vi "polling_mc.vi"() -> ()   [LabVIEW 2013, in "AvaSpec.lvlib" / "Avantes Spectrometer Functions.lvlib"]
uses:
  Avantes Spectrometer Functions.lvlib
  Instance          14 18Saved   polling_mc .vi
  Instance          13 18Saved   polling_mc .vi
  Instance          12 18Saved   polling_mc .vi
  Instance          10 18Saved   polling_mc .vi
  Instance           9 18Saved   polling_mc .vi
  Instance           8 18Saved   polling_mc .vi
panel:
  in  "a_pMeasConfig2":T1={"StartPixel"=0, "StopPixel"=0, "IntTime"=25.0, "IntDelay"=0, "NrOfAVG"=1, "DarkEnable"=0, "ForgetPercentage"=0, "SmoothPix"=0, "SmoothModel"=0, "SatDetection"=0, "TriggerMode"=0, "TriggerSource"=0, "TriggerSourceType"=0, "FlashesPerScan"=0, "LaserDelay"=0, "LaserWidth"=0, "LaserWavelenght"=0.0, "RamSpectra"=0}
  in  "a_pMeasConfig1":T1={"StartPixel"=0, "StopPixel"=0, "IntTime"=25.0, "IntDelay"=0, "NrOfAVG"=1, "DarkEnable"=0, "ForgetPercentage"=0, "SmoothPix"=0, "SmoothModel"=0, "SatDetection"=0, "TriggerMode"=0, "TriggerSource"=0, "TriggerSourceType"=0, "FlashesPerScan"=0, "LaserDelay"=0, "LaserWidth"=0, "LaserWavelenght"=0.0, "RamSpectra"=0}
  out "a_pNumPixels2":u16
  out "a_pNumPixels":u16
  in  "Sync Master":enum32{"Top Master", "Bottom Master"}(radio)
  in  "Sync Mode":enum32{"SyncMode On", "Sync Mode Off"}(radio)
  out "Serial2":string
  out "Serial1":string
  out "AVS_StopMeasure2":i32
  out "AVS_Deactivate2":i32
  out "Scope Values 2":cluster{"Y":dbl[], "Y":dbl[]}[](graph)
  out "a_pTimeLabel2":u32
  out "a_pDeviceId2":u8[](array[numeric])
  out "Handle2":i32
  out "Scope Values":cluster{"Y":dbl[], "Y":dbl[]}[](graph)
  out "a_pTimeLabel1":u32
  out "AVS_StopMeasure":i32
  out "AVS_Done":i32
  out "AVS_Deactivate":i32
  in  "Exit":bool
  in  "Stop":bool
  out "Handle1":i32
  out "a_pDeviceId1":u8[](array[numeric])
  in  "Start":bool
  in  "a_hWnd":i32
  out "Port":i32
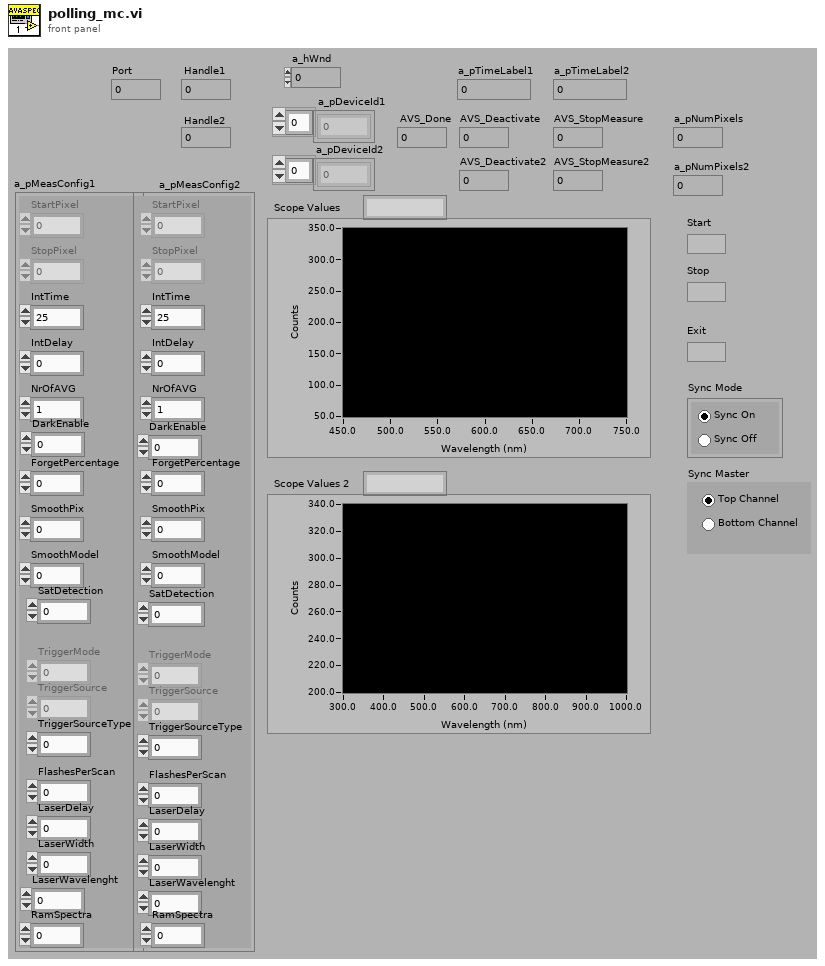
[diagram p1: front panel]
types:
  T1 = cluster{"StartPixel":u16, "StopPixel":u16, "IntTime":sgl, "IntDelay":u32, "NrOfAVG":u32, "DarkEnable":u8, "ForgetPercentage":u8, "SmoothPix":u16, "SmoothModel":u8, "SatDetection":u8, "TriggerMode":u8, "TriggerSource":u8, "TriggerSourceType":u8, "FlashesPerScan":u16, "LaserDelay":u32, "LaserWidth":u32, "LaserWavelenght":sgl, "RamSpectra":u16}
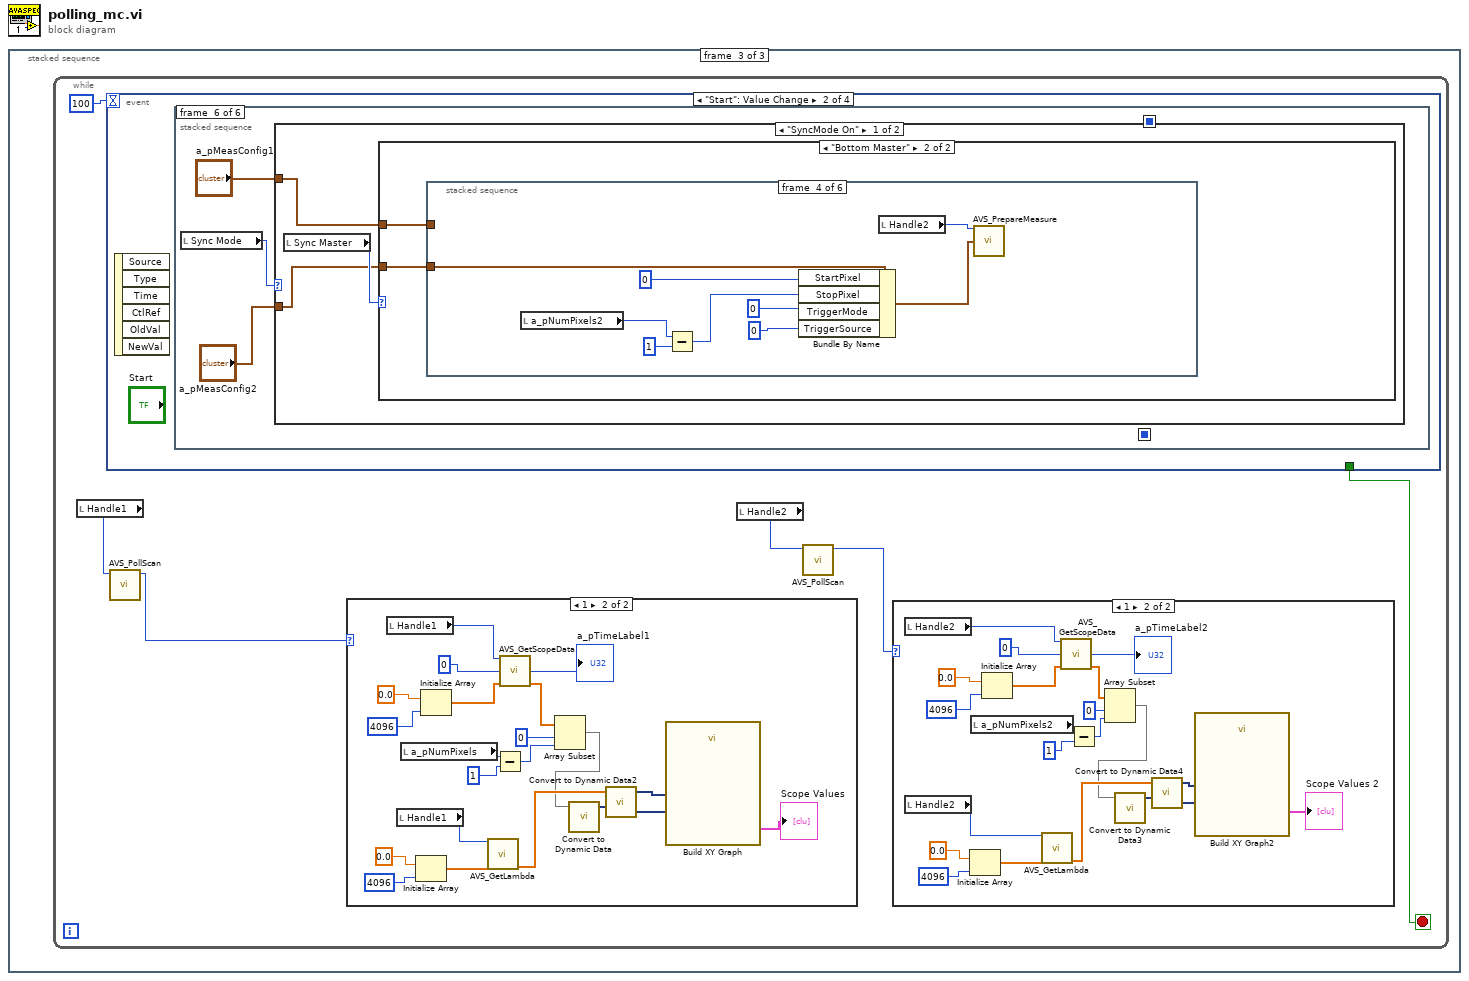
[diagram p0: block diagram]
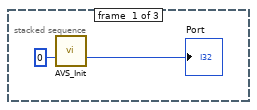
[diagram p2: hidden frame]
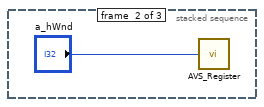
[diagram p3: hidden frame]
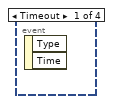
[diagram p6: hidden frame]
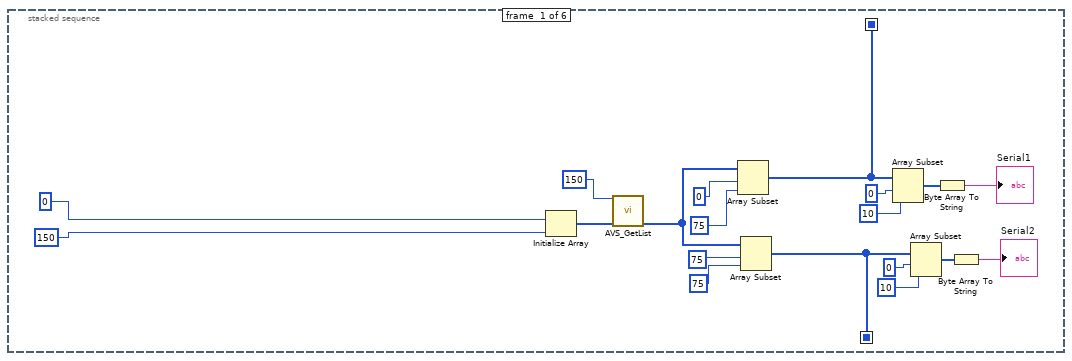
[diagram p7: hidden frame]
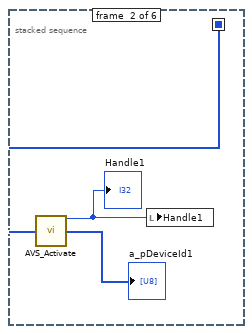
[diagram p8: hidden frame]
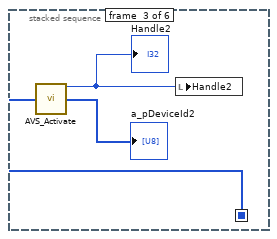
[diagram p9: hidden frame]
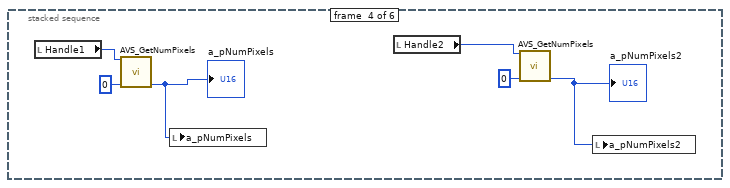
[diagram p10: hidden frame]
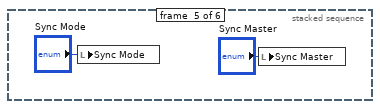
[diagram p11: hidden frame]
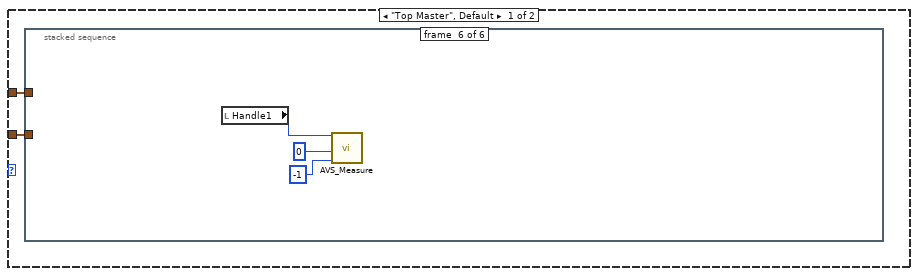
[diagram p12: hidden frame]
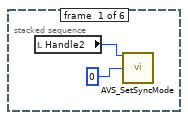
[diagram p13: hidden frame]
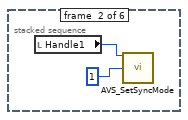
[diagram p14: hidden frame]
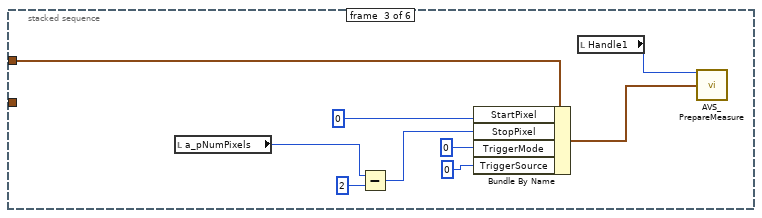
[diagram p15: hidden frame]
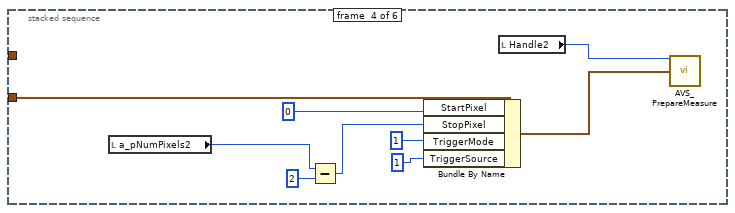
[diagram p16: hidden frame]
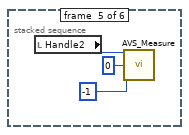
[diagram p17: hidden frame]
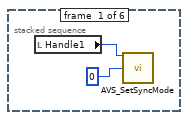
[diagram p18: hidden frame]
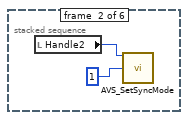
[diagram p19: hidden frame]
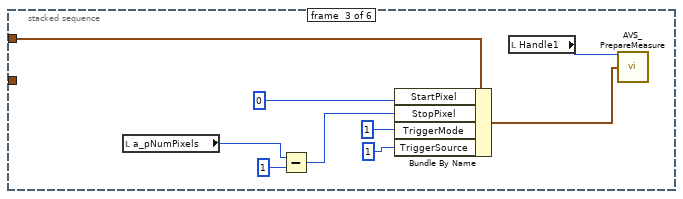
[diagram p20: hidden frame]
diagram:
  n1 = stacked-sequence {
    frame #0 {
      n2 = call "AVS_Init.vi"("a_Port"=0) -> ("Output Value"=→"Port":i32)  [unwired: 14 in]
    }
    frame #1 {
      n3 = call "AVS_Register.vi"("a_hWnd"="a_hWnd") -> ()  [unwired: 14 in, 1 out]
    }
    frame #2 {
      n4 = while {
        stop <- w8 stop-if-true
        n5 = local read "Handle1"() -> (w7:i32)
        n6 = event shown="[1] \"Start\": Value Change" {
          selector: _ -> [_ _ _ _]
          dyn-events: _ -> [_ _ _ _]
          timeout: 100 -> [_ _ _ _]
          tunnel: [_ _ _ "Exit"] -> w8
          event Timeout {
            n7 = event-data() -> ()  [unwired: 1 in, 2 out]
          }
          event "Start": Value Change {
            n8 = event-data() -> ()  [unwired: 1 in, 6 out]
            n9 = stacked-sequence {
              seq-local: [w57 _ _ _ _ _] -> [_ w69 _ _ _ _]
              seq-local: [w52 _ _ _ _ _] -> [_ _ w74 _ _ _]
              frame #0 {
                n10 = Initialize Array(i8 0 ("element"), 150 ("dimension size")) -> (w65:i8[])
                n11 = call "AVS_GetList.vi"("ListSizeInput"=u32 150, "ListInpit"=w65) -> ("List Output"=w64:u8[])  [unwired: 11 in, 2 out]
                n12 = Array Subset(array=w64, index=0, length=75) -> (w57:u8[])
                n13 = Array Subset(array=w64, index=75, length=75) -> (w52:u8[])
                n14 = Array Subset(array=w57, index=0, length=10) -> (w56:u8[])
                n15 = Array Subset(array=w52, index=0, length=10) -> (w51:u8[])
                n16 = Byte Array To String(unsigned byte array=w56) -> (string=→"Serial1":string)
                n17 = Byte Array To String(unsigned byte array=w51) -> (string=→"Serial2":string)
              }
              frame #1 {
                n18 = call "AVS_Activate.vi"("a_pDeviceId"=w69) -> ("Output Value"=w70:i32, "a_pDeviceId"=→"a_pDeviceId1":u8[])  [unwired: 13 in]
                "Handle1" <- w70
                n19 = local write "Handle1"(w70) -> ()
              }
              frame #2 {
                n20 = call "AVS_Activate.vi"("a_pDeviceId"=w74) -> ("Output Value"=w72:i32, "a_pDeviceId"=→"a_pDeviceId2":u8[])  [unwired: 13 in]
                "Handle2" <- w72
                n21 = local write "Handle2"(w72) -> ()
              }
              frame #3 {
                n22 = local read "Handle1"() -> (w80:i32)
                n23 = call "AVS_GetNumPixels.vi"("a_hDevice"=w80, "a_pNumPixels"=u16 0) -> ("a_pNumPixels"=w78:u16)  [unwired: 12 in, 1 out]
                "a_pNumPixels" <- w78
                n24 = local write "a_pNumPixels"(w78) -> ()
                n25 = local read "Handle2"() -> (w77:i32)
                n26 = call "AVS_GetNumPixels.vi"("a_hDevice"=w77, "a_pNumPixels"=u16 0) -> ("a_pNumPixels"=w75:u16)  [unwired: 12 in, 1 out]
                "a_pNumPixels2" <- w75
                n27 = local write "a_pNumPixels2"(w75) -> ()
              }
              frame #4 {
                n28 = local write "Sync Mode"("Sync Mode") -> ()
                n29 = local write "Sync Master"("Sync Master") -> ()
              }
              frame #5 {
                n30 = local read "Sync Mode"() -> (w85:enum32{"SyncMode On", "Sync Mode Off"})
                n31 = case shown="\"SyncMode On\"" w85 {
                  tunnel: "a_pMeasConfig1" -> [w87 w150]
                  tunnel: "a_pMeasConfig2" -> [w86 w149]
                  frame "SyncMode On" {
                    n32 = local read "Sync Master"() -> (w88:enum32{"Top Master", "Bottom Master"})
                    n33 = case shown="\"Bottom Master\"" w88 {
                      tunnel: w87 -> [w90 w120]
                      tunnel: w86 -> [w89 w119]
                      frame "Top Master", Default {
                        n34 = stacked-sequence {
                          tunnel: w90 -> [_ _ w97 _ _ _]
                          tunnel: w89 -> [_ _ _ w106 _ _]
                          frame #0 {
                            n35 = local read "Handle2"() -> (w91:i32)
                            n36 = call "AVS_SetSyncMode.vi"("a_hDevice"=w91, "a_Enable"=u8 0) -> ()  [unwired: 13 in, 1 out]
                          }
                          frame #1 {
                            n37 = local read "Handle1"() -> (w93:i32)
                            n38 = call "AVS_SetSyncMode.vi"("a_hDevice"=w93, "a_Enable"=u8 1) -> ()  [unwired: 13 in, 1 out]
                          }
                          frame #2 {
                            n39 = local read "a_pNumPixels"() -> (w95:u16)
                            n40 = Subtract(x=w95, y=u16 2) -> (x-y=w100:u16)
                            n41 = Bundle By Name(cluster=w97, "StartPixel"=0, "StopPixel"=w100, "TriggerMode"=u8 0, "TriggerSource"=u8 0) -> (w96:T1)
                            n42 = local read "Handle1"() -> (w103:i32)
                            n43 = call "AVS_PrepareMeasure.vi"("a_hDevice"=w103, "a_pMeasConfig"=w96) -> ()  [unwired: 13 in, 1 out]
                          }
                          frame #3 {
                            n44 = local read "a_pNumPixels2"() -> (w109:u16)
                            n45 = Subtract(x=w109, y=u16 2) -> (x-y=w107:u16)
                            n46 = Bundle By Name(cluster=w106, "StartPixel"=0, "StopPixel"=w107, "TriggerMode"=u8 1, "TriggerSource"=u8 1) -> (w105:T1)
                            n47 = local read "Handle2"() -> (w104:i32)
                            n48 = call "AVS_PrepareMeasure.vi"("a_hDevice"=w104, "a_pMeasConfig"=w105) -> ()  [unwired: 13 in, 1 out]
                          }
                          frame #4 {
                            n49 = local read "Handle2"() -> (w115:i32)
                            n50 = call "AVS_Measure.vi"("a_hDevice"=w115, "a_hWnd"=0, "a_Nmsr"=i16 -1) -> ()  [unwired: 12 in, 1 out]
                          }
                          frame #5 {
                            n51 = local read "Handle1"() -> (w116:i32)
                            n52 = call "AVS_Measure.vi"("a_hDevice"=w116, "a_hWnd"=0, "a_Nmsr"=i16 -1) -> ()  [unwired: 12 in, 1 out]
                          }
                        }
                      }
                      frame "Bottom Master" {
                        n53 = stacked-sequence {
                          tunnel: w120 -> [_ _ w129 _ _ _]
                          tunnel: w119 -> [_ _ _ w137 _ _]
                          frame #0 {
                            n54 = local read "Handle1"() -> (w121:i32)
                            n55 = call "AVS_SetSyncMode.vi"("a_hDevice"=w121, "a_Enable"=u8 0) -> ()  [unwired: 13 in, 1 out]
                          }
                          frame #1 {
                            n56 = local read "Handle2"() -> (w123:i32)
                            n57 = call "AVS_SetSyncMode.vi"("a_hDevice"=w123, "a_Enable"=u8 1) -> ()  [unwired: 13 in, 1 out]
                          }
                          frame #2 {
                            n58 = local read "a_pNumPixels"() -> (w128:u16)
                            n59 = Subtract(x=w128, y=u16 1) -> (x-y=w132:u16)
                            n60 = Bundle By Name(cluster=w129, "StartPixel"=0, "StopPixel"=w132, "TriggerMode"=u8 1, "TriggerSource"=u8 1) -> (w125:T1)
                            n61 = local read "Handle1"() -> (w126:i32)
                            n62 = call "AVS_PrepareMeasure.vi"("a_hDevice"=w126, "a_pMeasConfig"=w125) -> ()  [unwired: 13 in, 1 out]
                          }
                          frame #3 {
                            n63 = local read "a_pNumPixels2"() -> (w136:u16)
                            n64 = Subtract(x=w136, y=u16 1) -> (x-y=w140:u16)
                            n65 = Bundle By Name(cluster=w137, "StartPixel"=0, "StopPixel"=w140, "TriggerMode"=u8 0, "TriggerSource"=u8 0) -> (w134:T1)
                            n66 = local read "Handle2"() -> (w135:i32)
                            n67 = call "AVS_PrepareMeasure.vi"("a_hDevice"=w135, "a_pMeasConfig"=w134) -> ()  [unwired: 13 in, 1 out]
                          }
                          frame #4 {
                            n68 = local read "Handle1"() -> (w145:i32)
                            n69 = call "AVS_Measure.vi"("a_hDevice"=w145, "a_hWnd"=0, "a_Nmsr"=i16 -1) -> ()  [unwired: 12 in, 1 out]
                          }
                          frame #5 {
                            n70 = local read "Handle2"() -> (w146:i32)
                            n71 = call "AVS_Measure.vi"("a_hDevice"=w146, "a_hWnd"=0, "a_Nmsr"=i16 -1) -> ()  [unwired: 12 in, 1 out]
                          }
                        }
                      }
                    }
                  }
                  frame "Sync Mode Off" {
                    n72 = stacked-sequence {
                      tunnel: w150 -> [_ _ w155 _ _ _]
                      tunnel: w149 -> [_ _ _ w164 _ _]
                      frame #0 {
                        n73 = local read "Handle1"() -> (w151:i32)
                        n74 = call "AVS_SetSyncMode.vi"("a_hDevice"=w151, "a_Enable"=u8 0) -> ()  [unwired: 13 in, 1 out]
                      }
                      frame #1 {
                        n75 = local read "Handle2"() -> (w153:i32)
                        n76 = call "AVS_SetSyncMode.vi"("a_hDevice"=w153, "a_Enable"=u8 0) -> ()  [unwired: 13 in, 1 out]
                      }
                      frame #2 {
                        n77 = local read "a_pNumPixels"() -> (w160:u16)
                        n78 = Subtract(x=w160, y=u16 2) -> (x-y=w158:u16)
                        n79 = Bundle By Name(cluster=w155, "StartPixel"=0, "StopPixel"=w158, "TriggerMode"=u8 0, "TriggerSource"=u8 0) -> (w162:T1)
                        n80 = local read "Handle1"() -> (w163:i32)
                        n81 = call "AVS_PrepareMeasure.vi"("a_hDevice"=w163, "a_pMeasConfig"=w162) -> ()  [unwired: 13 in, 1 out]
                      }
                      frame #3 {
                        n82 = local read "a_pNumPixels2"() -> (w166:u16)
                        n83 = Subtract(x=w166, y=u16 2) -> (x-y=w169:u16)
                        n84 = Bundle By Name(cluster=w164, "StartPixel"=0, "StopPixel"=w169, "TriggerMode"=u8 0, "TriggerSource"=u8 0) -> (w165:T1)
                        n85 = local read "Handle2"() -> (w172:i32)
                        n86 = call "AVS_PrepareMeasure.vi"("a_hDevice"=w172, "a_pMeasConfig"=w165) -> ()  [unwired: 13 in, 1 out]
                      }
                      frame #4 {
                        n87 = local read "Handle1"() -> (w175:i32)
                        n88 = call "AVS_Measure.vi"("a_hDevice"=w175, "a_hWnd"=0, "a_Nmsr"=i16 -1) -> ()  [unwired: 12 in, 1 out]
                      }
                      frame #5 {
                        n89 = local read "Handle2"() -> (w176:i32)
                        n90 = call "AVS_Measure.vi"("a_hDevice"=w176, "a_hWnd"=0, "a_Nmsr"=i16 -1) -> ()  [unwired: 12 in, 1 out]
                      }
                    }
                  }
                }
              }
            }
          }
          event "Stop": Value Change {
            n91 = event-data() -> ()  [unwired: 1 in, 6 out]
            n92 = stacked-sequence {
              frame #0 {
                n93 = local read "Handle1"() -> (w180:i32)
                n94 = call "AVS_StopMeasure.vi"("a_hDevice"=w180) -> ("Output Value"=→"AVS_StopMeasure":i32)  [unwired: 14 in]
              }
              frame #1 {
                n95 = local read "Handle2"() -> (w181:i32)
                n96 = call "AVS_StopMeasure.vi"("a_hDevice"=w181) -> ("Output Value"=→"AVS_StopMeasure2":i32)  [unwired: 14 in]
              }
              frame #2 {
                n97 = local read "Handle1"() -> (w184:i32)
                n98 = call "AVS_Deactivate.vi"("a_hHandle"=w184) -> ("Output Value"=→"AVS_Deactivate":i32)  [unwired: 14 in]
              }
              frame #3 {
                n99 = local read "Handle2"() -> (w185:i32)
                n100 = call "AVS_Deactivate.vi"("a_hHandle"=w185) -> ("Output Value"=→"AVS_Deactivate2":i32)  [unwired: 14 in]
              }
            }
          }
          event "Exit": Value Change {
            n101 = event-data() -> ()  [unwired: 1 in, 6 out]
            n102 = call "AVS_Done.vi"() -> ("Output Value"=→"AVS_Done":i32)  [unwired: 19 in]
          }
        }
        n103 = call "AVS_PollScan.vi"("a_hDevice"=w7) -> ("Output Value"=w6:i32)  [unwired: 8 in]
        n104 = case shown="1" w6 {
          frame 0, Default {
          }
          frame 1 {
            n105 = local read "Handle1"() -> (w46:i32)
            n106 = local read "Handle1"() -> (w41:i32)
            n107 = local read "a_pNumPixels"() -> (w34:u16)
            n108 = Initialize Array(0.0 ("element"), 4096 ("dimension size")) -> (w40:dbl[])
            n109 = Initialize Array(0.0 ("element"), 4096 ("dimension size")) -> (w49:dbl[])
            n110 = call "AVS_GetLambda.vi"("a_hDevice"=w41, "a_pWaveLength"=w40) -> ("a_pWaveLength"=w37:dbl[])  [unwired: 12 in, 1 out]
            n111 = Subtract(x=w34, y=u16 1) -> (x-y=w33:u16)
            n112 = call "AVS_GetScopeData.vi"("a_hDevice"=w46, "a_pTimeLabel"=0, "a_pSpectrum"=w49) -> ("a_pTimeLabel"=→"a_pTimeLabel1":u32, "a_pSpectrum"=w31:dbl[])  [unwired: 10 in, 1 out]
            n113 = Array Subset(array=w31, index=0, length=w33) -> (w30:dbl[])
            n114 = call "Convert to Dynamic Data"("Array"=w30) -> ("Dynamic Data Type"=w43:dynamicdata)  [unwired: 3 in]
            n115 = call "Convert to Dynamic Data2"("Array"=w37) -> ("Dynamic Data Type"=w42:dynamicdata)  [unwired: 3 in]
            n116 = call "Build XY Graph"("Y Input"=w43, "X Input"=w42) -> ("XY Graph"=→"Scope Values":cluster{"Y":dbl[], "Y":dbl[]}[])  [unwired: 8 in, 1 out]
          }
        }
        n117 = local read "Handle2"() -> (w5:i32)
        n118 = call "AVS_PollScan.vi"("a_hDevice"=w5) -> ("Output Value"=w4:i32)  [unwired: 8 in]
        n119 = case shown="1" w4 {
          frame 0, Default {
          }
          frame 1 {
            n120 = local read "Handle2"() -> (w25:i32)
            n121 = local read "Handle2"() -> (w21:i32)
            n122 = Initialize Array(0.0 ("element"), 4096 ("dimension size")) -> (w24:dbl[])
            n123 = local read "a_pNumPixels2"() -> (w14:u16)
            n124 = Initialize Array(0.0 ("element"), 4096 ("dimension size")) -> (w29:dbl[])
            n125 = call "AVS_GetLambda.vi"("a_hDevice"=w21, "a_pWaveLength"=w24) -> ("a_pWaveLength"=w17:dbl[])  [unwired: 12 in, 1 out]
            n126 = call "AVS_GetScopeData.vi"("a_hDevice"=w25, "a_pTimeLabel"=0, "a_pSpectrum"=w29) -> ("a_pTimeLabel"=→"a_pTimeLabel2":u32, "a_pSpectrum"=w11:dbl[])  [unwired: 10 in, 1 out]
            n127 = Subtract(x=w14, y=u16 1) -> (x-y=w13:u16)
            n128 = Array Subset(array=w11, index=0, length=w13) -> (w10:dbl[])
            n129 = call "Convert to Dynamic Data3"("Array"=w10) -> ("Dynamic Data Type"=w20:dynamicdata)  [unwired: 3 in]
            n130 = call "Convert to Dynamic Data4"("Array"=w17) -> ("Dynamic Data Type"=w19:dynamicdata)  [unwired: 3 in]
            n131 = call "Build XY Graph2"("Y Input"=w20, "X Input"=w19) -> ("XY Graph"=→"Scope Values 2":cluster{"Y":dbl[], "Y":dbl[]}[])  [unwired: 8 in, 1 out]
          }
        }
      }
    }
  }
